vi "CIEncoderProps.vi"(0 "task in":refnum<k24>, 3 "error in (no error)":errorcluster) -> (4 "Units":i32, 5 "DecodingType":i32, 6 "task out":refnum<k24>, 7 "PulsesPerRevolution":i32, 8 "InitialAngle":dbl, 9 "ZIndexMode":i32, 10 "error out":errorcluster)   [LabVIEW 2010]
uses:
  C:/Program Files/National Instruments/LabVIEW 2010/vi.lib/ULx/ULx_LV.dll
  Program Files/National Instruments/LabVIEW 2010/vi.lib/ULx/ULx_LV.dll
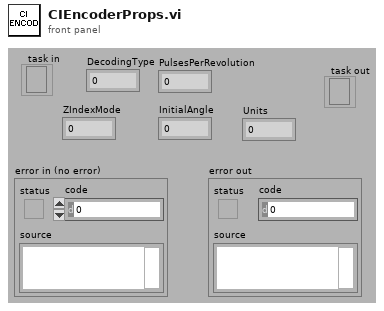
[diagram p1: front panel]
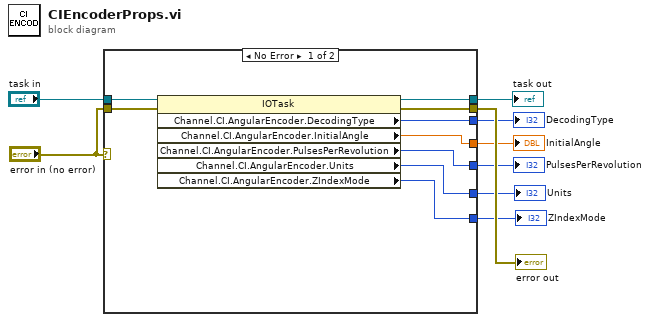
[diagram p0: block diagram]
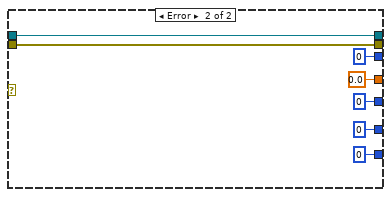
[diagram p2: hidden frame]
diagram:
  n1 = case shown="No Error" "error in (no error)" {
    tunnel: "task in" -> [w18 w25]
    tunnel: "error in (no error)" -> [w17 w24]
    tunnel: [w16 w25] -> w8
    tunnel: [w15 w24] -> w7
    tunnel: [w14 0 ("Channel.CI.AngularEncoder.DecodingType")] -> w5
    tunnel: [w13 0.0 ("Channel.CI.AngularEncoder.InitialAngle")] -> w4
    tunnel: [w12 0 ("Channel.CI.AngularEncoder.PulsesPerRevolution")] -> w3
    tunnel: [w11 0 ("Channel.CI.AngularEncoder.Units")] -> w2
    tunnel: [w10 0 ("Channel.CI.AngularEncoder.ZIndexMode")] -> w1
    frame No Error {
      n2 = property class="IOTask"(reference=w18, error in=w17) -> (reference out=w16:refnum<k24>, error out=w15:errorcluster, "Channel.CI.AngularEncoder.DecodingType"=w14:i32, "Channel.CI.AngularEncoder.InitialAngle"=w13:dbl, "Channel.CI.AngularEncoder.PulsesPerRevolution"=w12:i32, "Channel.CI.AngularEncoder.Units"=w11:i32, "Channel.CI.AngularEncoder.ZIndexMode"=w10:i32)
    }
    frame Error {
    }
  }
  "task out" <- w8
  "error out" <- w7
  "DecodingType" <- w5
  "InitialAngle" <- w4
  "PulsesPerRevolution" <- w3
  "Units" <- w2
  "ZIndexMode" <- w1
